vi "20TVTI_Set_Monitor_Values.vi"(3 "VTI Status":T1={"Temperatur (K)"=70.6986, "Heater (%)"=0.0017142857142857142, "NV (%)"=0.0, "Heater Manual"=TRUE, "NV Manual"=TRUE, "Pressure"=1.0208606, "Dewar Pressure"=1.0500276, "Valid?"=FALSE, "Dewar Heater Manual"=FALSE, "Heater (%) Display"=0.0, "NV (%) Display"=0.0, "Dewar Heater (%)"=18.434412358753207, "D-Heater (%) Display"=18.434412358753207} {"Heater (%)" scale=0.0..100.0; "NV (%)" scale=0.0..100.0; "Dewar Heater (%)" scale=0.0..100.0}, 5 "System Monitor Variables (in)":T2) -> (1 "System Monitor Variables (out)":T2)   [LabVIEW 2016]
uses:
  Global/Global Variables/System Monitor Cluster.ctl
  Gustav/20TVTI_Status.ctl
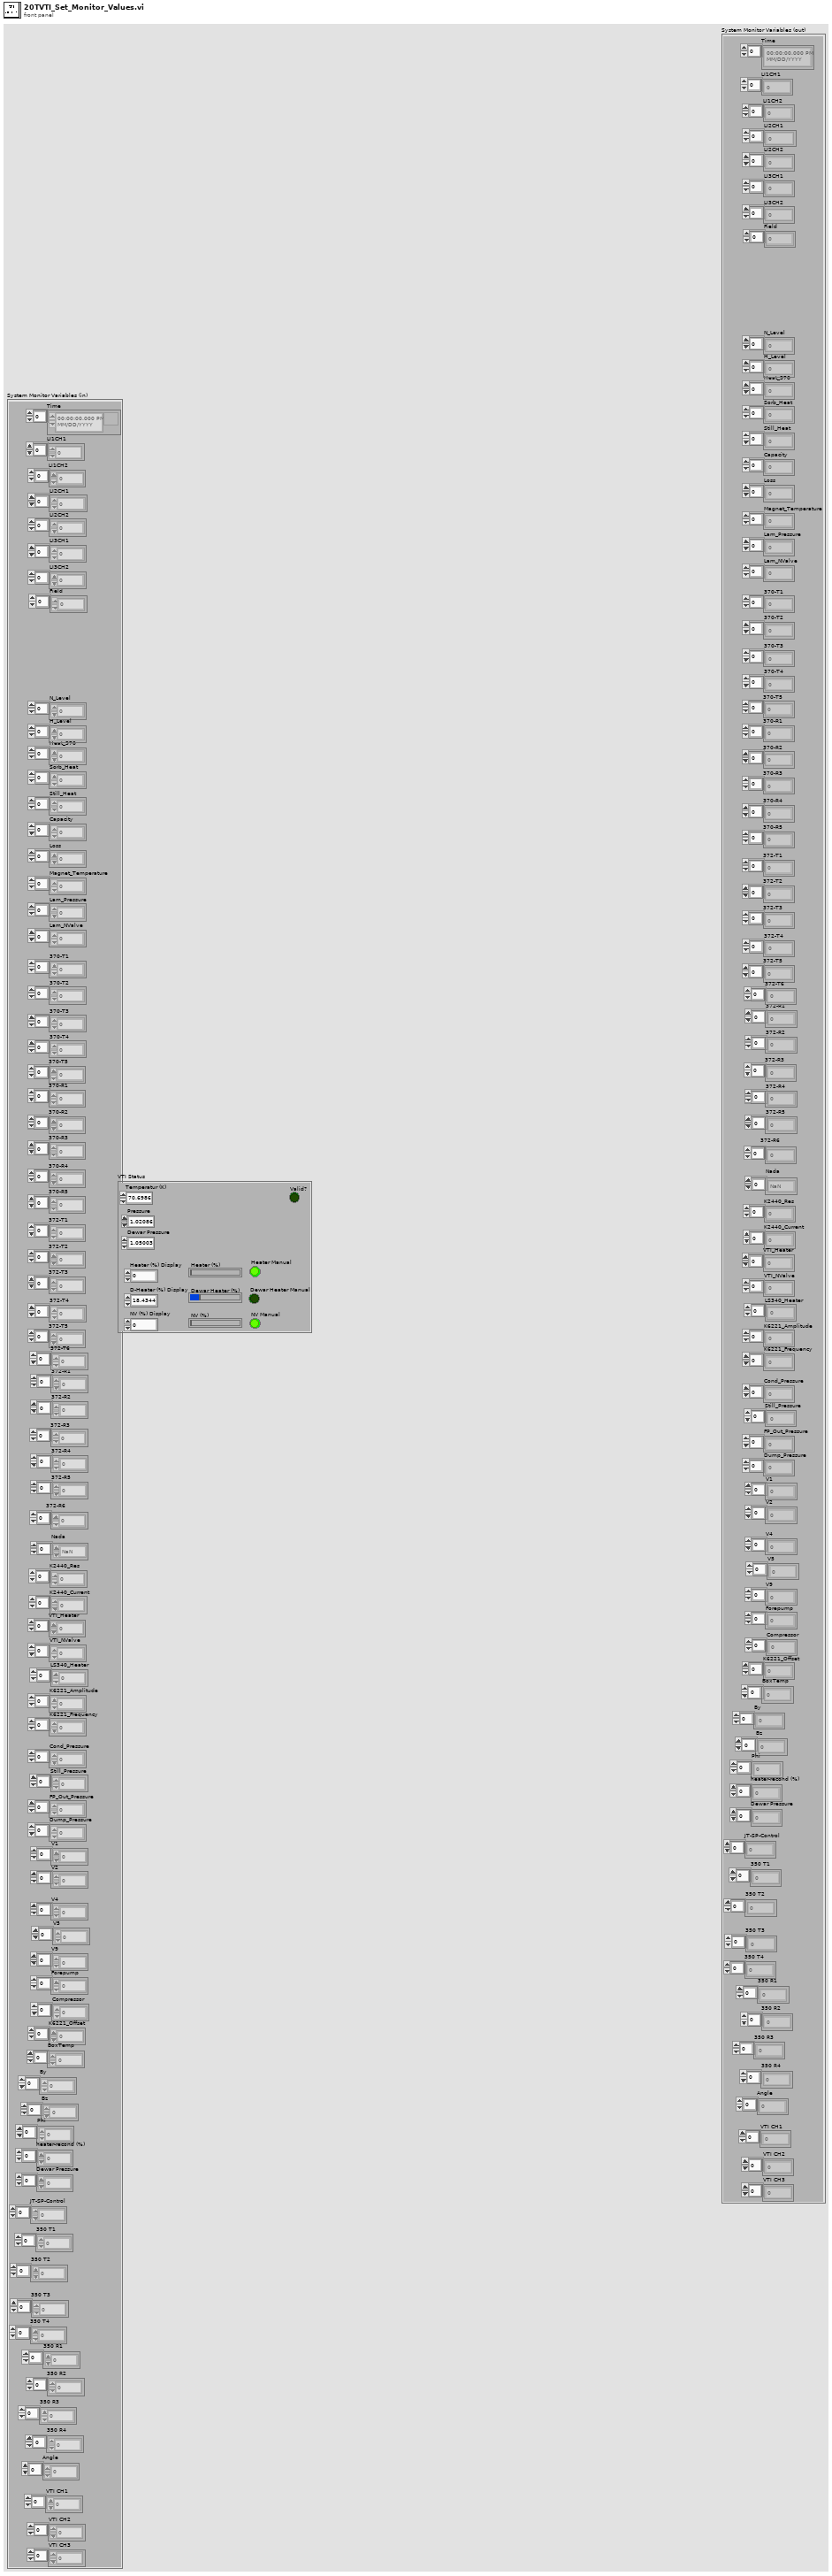
[diagram p1: front panel]
types:
  T1 = typedef "20TVTI_Status.ctl" = cluster{"Temperatur (K)":dbl, "Heater (%)":dbl, "NV (%)":dbl, "Heater Manual":bool, "NV Manual":bool, "Pressure":dbl, "Dewar Pressure":dbl, "Valid?":bool, "Dewar Heater Manual":bool, "Heater (%) Display":dbl, "NV (%) Display":dbl, "Dewar Heater (%)":dbl, "D-Heater (%) Display":dbl}
  T2 = typedef "System Monitor Cluster.ctl" = cluster{"Time":timestamp[], "LI1CH1":dbl[], "LI1CH2":dbl[], "LI2CH1":dbl[], "LI2CH2":dbl[], "LI3CH1":dbl[], "LI3CH2":dbl[], "Field":dbl[], "N_Level":dbl[], "H_Level":dbl[], "Heat_370":dbl[], "Sorb_Heat":dbl[], "Still_Heat":dbl[], "Capacity":dbl[], "Loss":dbl[], "Magnet_Temperature":dbl[], "Lam_Pressure":dbl[], "Lam_NValve":dbl[], "370-T1":dbl[], "370-T2":dbl[], "370-T3":dbl[], "370-T4":dbl[], "370-T5":dbl[], "370-R1":dbl[], "370-R2":dbl[], "370-R3":dbl[], "370-R4":dbl[], "370-R5":dbl[], "372-T1":dbl[], "372-T2":dbl[], "372-T3":dbl[], "372-T4":dbl[], "372-T5":dbl[], "372-T6":dbl[], "372-R1":dbl[], "372-R2":dbl[], "372-R3":dbl[], "372-R4":dbl[], "372-R5":dbl[], "372-R6":dbl[], "Nada":dbl[], "K2440_Res":dbl[], "K2440_Current":dbl[], "VTI_Heater":dbl[], "VTI_NValve":dbl[], "LS340_Heater":dbl[], "K6221_Amplitude":dbl[], "K6221_Frequency":dbl[], "Cond_Pressure":dbl[], "Still_Pressure":dbl[], "FP_Out_Pressure":dbl[], "Dump_Pressure":dbl[], "V1":dbl[], "V2":dbl[], "V4":dbl[], "V5":dbl[], "V9":dbl[], "Forepump":dbl[], "Compressor":dbl[], "K6221_Offset":dbl[], "BoxTemp":dbl[], "By":dbl[], "Bz":dbl[], "Phi":dbl[], "heater-recond (%)":dbl[], "Dewar Pressure ":dbl[], "JT-SP-Control":dbl[], "350 T1":dbl[], "350 T2":dbl[], "350 T3":dbl[], "350 T4":dbl[], "350 R1":dbl[], "350 R2":dbl[], "350 R3":dbl[], "350 R4":dbl[], "Angle":dbl[], "VTI CH1":dbl[], "VTI CH2":dbl[], "VTI CH3":dbl[]}
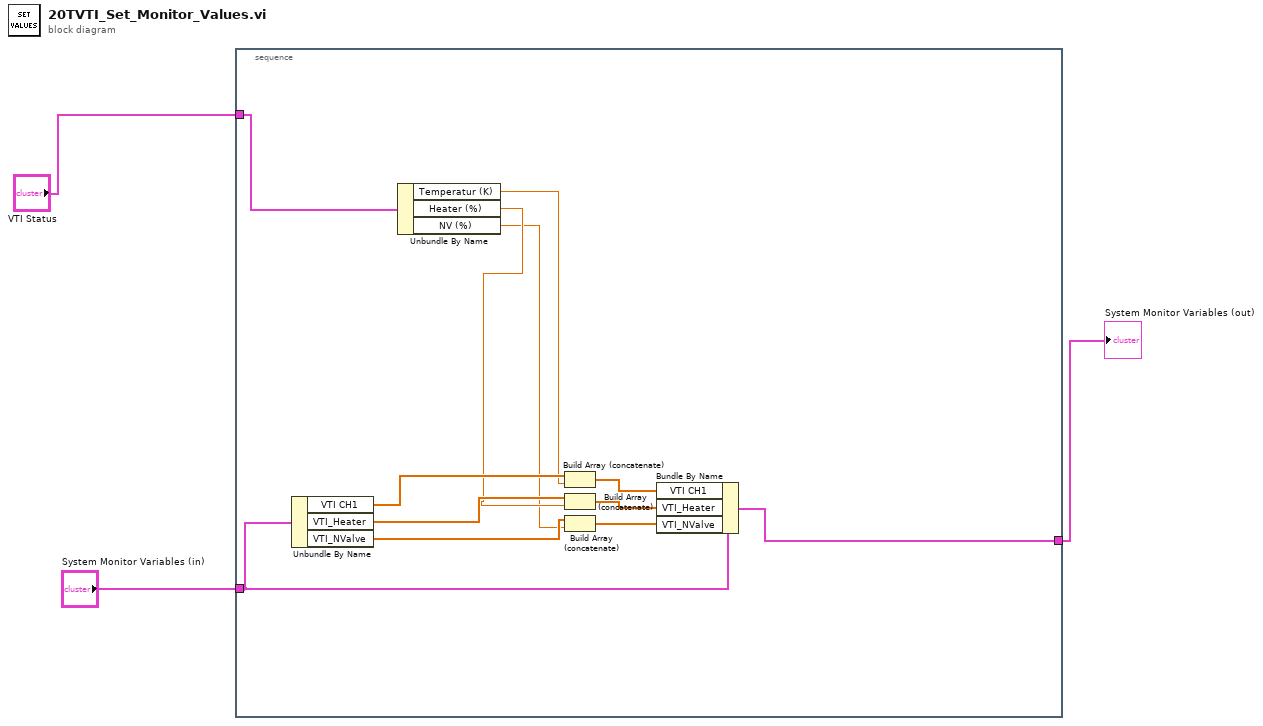
[diagram p0: block diagram]
diagram:
  n1 = stacked-sequence {
    tunnel: "System Monitor Variables (in)" -> [w5]
    tunnel: [w9] -> w2
    tunnel: "VTI Status" -> [w4]
    frame #0 {
      n2 = Unbundle By Name(w5) -> ("VTI CH1"=w15:dbl[], "VTI_Heater"=w14:dbl[], "VTI_NValve"=w13:dbl[])
      n3 = Unbundle By Name(w4) -> ("Temperatur (K)"=w12:dbl, "Heater (%)"=w11:dbl, "NV (%)"=w10:dbl)
      n4 = Build Array (concatenate)(w15, w12) -> (w8:dbl[])
      n5 = Build Array (concatenate)(w14, w11) -> (w7:dbl[])
      n6 = Build Array (concatenate)(w13, w10) -> (w6:dbl[])
      n7 = Bundle By Name(cluster=w5, "VTI CH1"=w8, "VTI_Heater"=w7, "VTI_NValve"=w6) -> (w9:T2)
    }
  }
  "System Monitor Variables (out)" <- w2
